vi "Traverse_Space_Server.vi"(6 "Probe Support":T1=[{"Max"=15.0, "Min"=-15.0}, {"Max"=250.0, "Min"=0.0}, {"Max"=15.0, "Min"=-15.0}] {"Min" format="%#.1f"; "Max" format="%#.1f"}, 7 "Mode":T4(ring), 8 "Entire Space":T1=[{"Max"=15001.0, "Min"=12000.0}, {"Max"=1000.0, "Min"=-1000.0}, {"Max"=700.0, "Min"=0.0}] {"Min" format="%#.1f"; "Max" format="%#.1f"}, 9 "Probe Volume":T1=[{"Max"=0.0, "Min"=0.0}, {"Max"=250.0, "Min"=0.0}, {"Max"=15.0, "Min"=-15.0}] {"Min" format="%#.1f"; "Max" format="%#.1f"}, 10 "Exclude Array":T2[](array[typedef]) {"Sizes"."Min" format="%#.1f"; "Sizes"."Max" format="%#.1f"}, 11 "Traverse Name":string) -> (0 "Entire Space Out":T1=[{"Max"=15001.0, "Min"=12000.0}, {"Max"=1000.0, "Min"=-1000.0}, {"Max"=700.0, "Min"=0.0}] {"Min" format="%#.1f"; "Max" format="%#.1f"}, 1 "Probe Volume Out":T1=[{"Max"=15.0, "Min"=-15.0}, {"Max"=250.0, "Min"=0.0}, {"Max"=15.0, "Min"=-15.0}] {"Min" format="%#.1f"; "Max" format="%#.1f"}, 2 "Exclude Array Out":T2[](array[typedef])=[{"Sizes"=[{"Max"=15000.0, "Min"=0.0}, {"Max"=1000.0, "Min"=-1000.0}, {"Max"=300.0, "Min"=0.0}], "Name"="Roughness Elements", "Exclude Type"=enum."Allow only vertical moves"}, {"Sizes"=[{"Max"=17000.0, "Min"=16000.0}, {"Max"=200.0, "Min"=-200.0}, {"Max"=-50.0, "Min"=-250.0}], "Name"="B204", "Exclude Type"=enum."Exclude completely"}] {"Sizes"."Min" format="%#.1f"; "Sizes"."Max" format="%#.1f"}, 3 "Error Comments":string, 4 "Probe Support Out":T1=[{"Max"=15.0, "Min"=-15.0}, {"Max"=250.0, "Min"=0.0}, {"Max"=15.0, "Min"=-15.0}] {"Min" format="%#.1f"; "Max" format="%#.1f"}, 5 "Space File":path)   [LabVIEW 2013]
uses:
  Gen Trav/Route mapping/Exclude_cluster.ctl
  Gen Trav/Route mapping/Box_size.ctl
  Gen Trav/Route mapping/Exclusion_type.ctl
  Globals/Constants_global.vi
panel:
  in  "Row type":string
  in  "Integer":i32
  out "Channel Values":string[][](array[string])
  # "(Relative to measurement position)"
  # "X                           Y                          Z"
  # "(Relative to measurement position)"
  # "X                           Y                          Z"
  # "X                           Y                          Z"
  # "X                           Y                          Z"
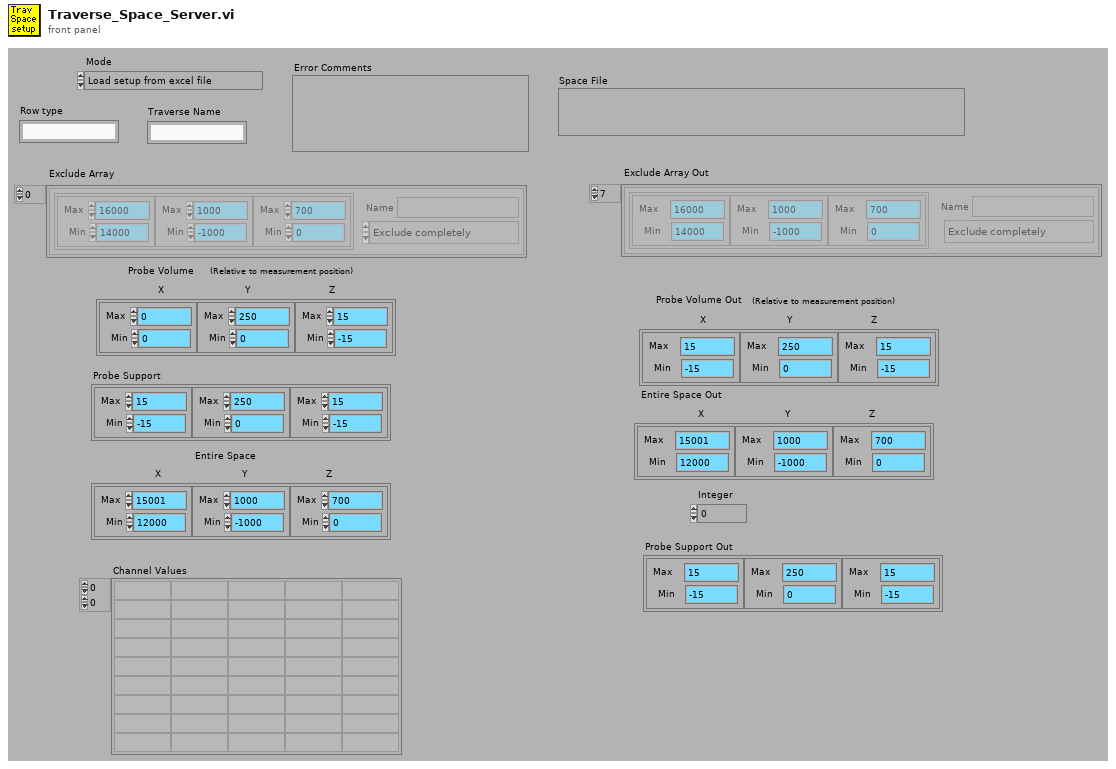
[diagram p1: front panel]
types:
  T1 = typedef "Box_size.ctl" = cluster{"Max":dbl, "Min":dbl}[]
  T2 = typedef "Exclude_cluster.ctl" = cluster{"Sizes":T1, "Name":string, "Exclude Type":T3}
  T3 = typedef "Exclusion_type.ctl" = enum16{"Exclude completely", "Allow only vertical moves"}
  T4 = enum16{"Load setup from excel file", "Save setup to excel file"}
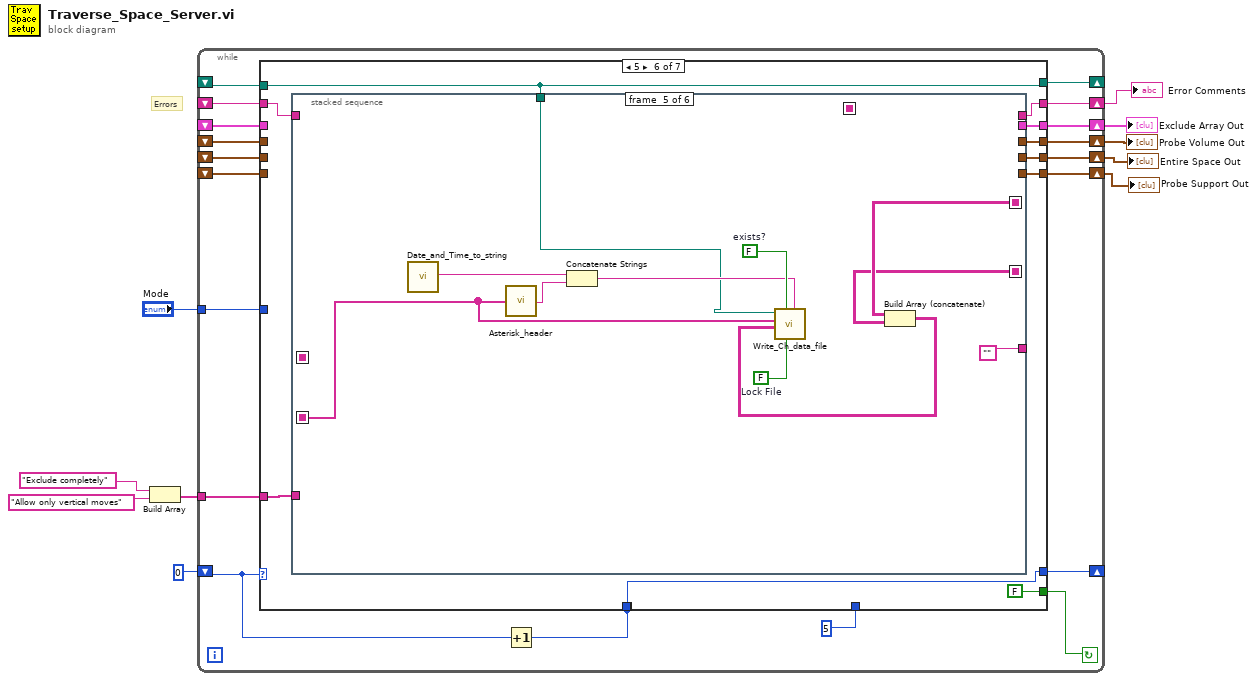
[diagram p0: block diagram]
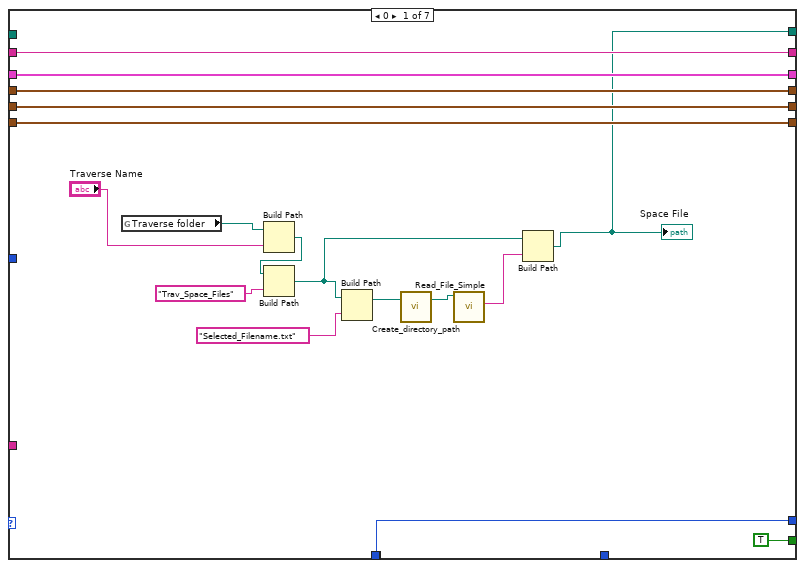
[diagram p2: hidden frame]
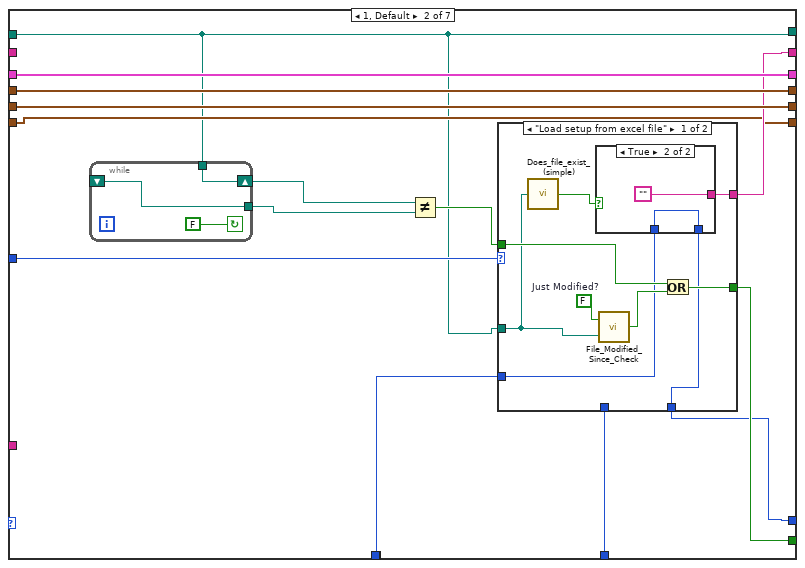
[diagram p3: hidden frame]
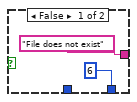
[diagram p4: hidden frame]
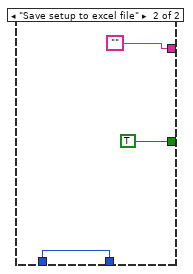
[diagram p5: hidden frame]
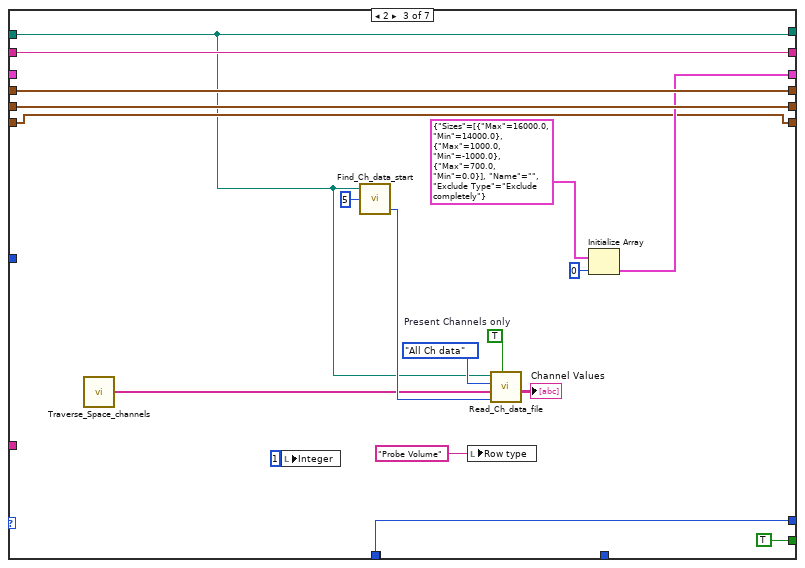
[diagram p6: hidden frame]
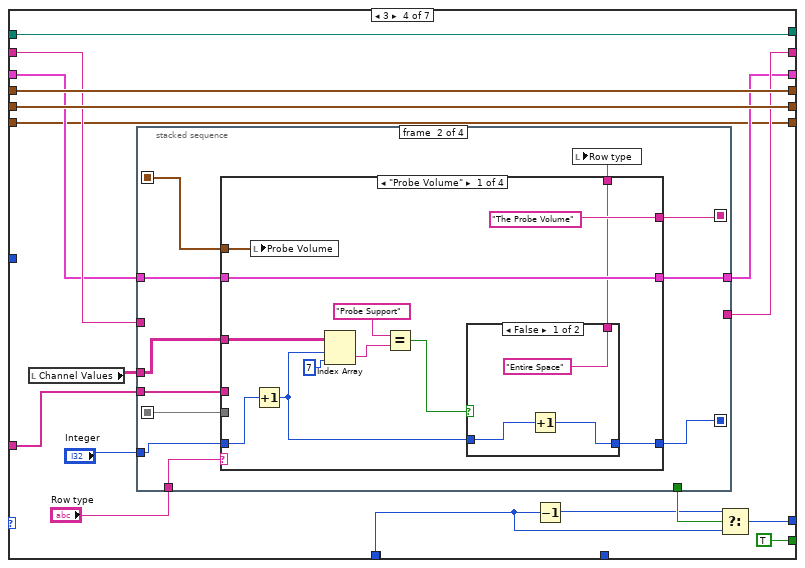
[diagram p7: hidden frame]
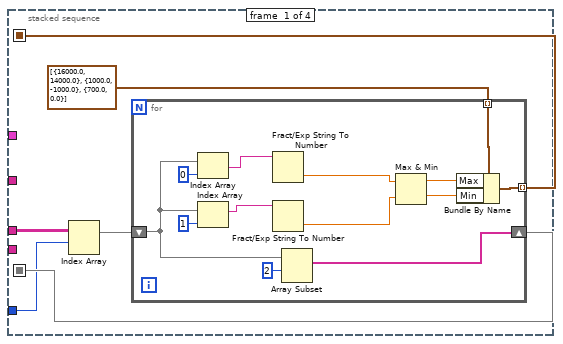
[diagram p8: hidden frame]
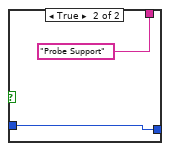
[diagram p9: hidden frame]
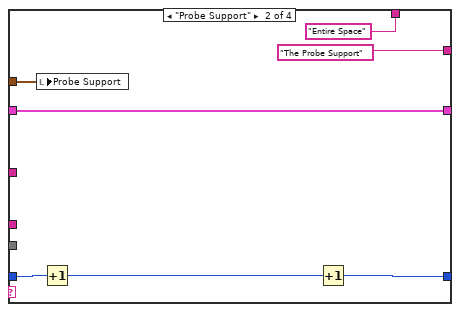
[diagram p10: hidden frame]
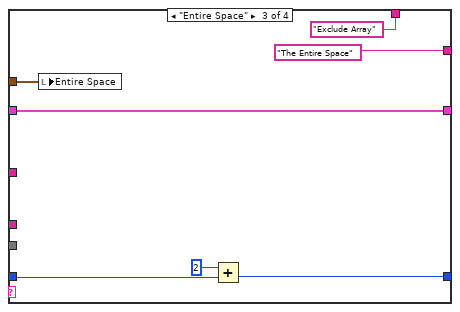
[diagram p11: hidden frame]
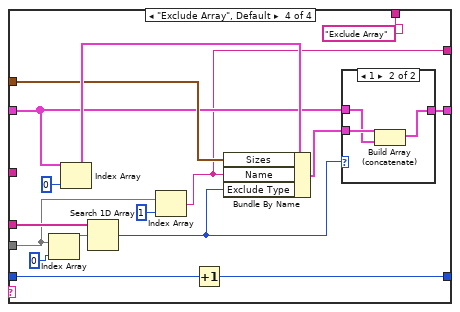
[diagram p12: hidden frame]
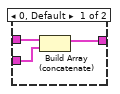
[diagram p13: hidden frame]
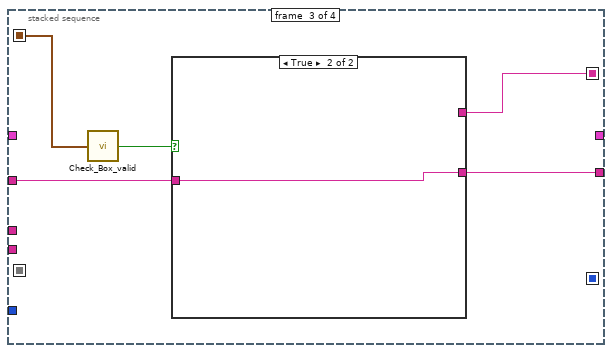
[diagram p14: hidden frame]
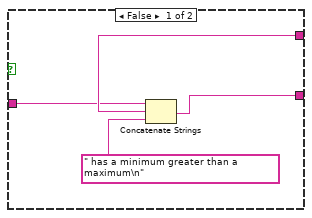
[diagram p15: hidden frame]
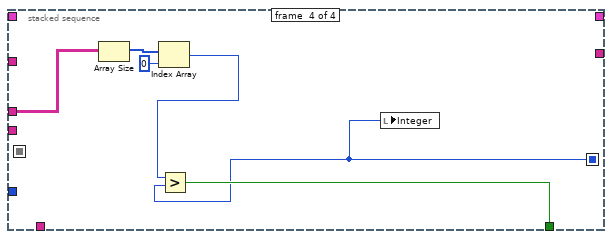
[diagram p16: hidden frame]
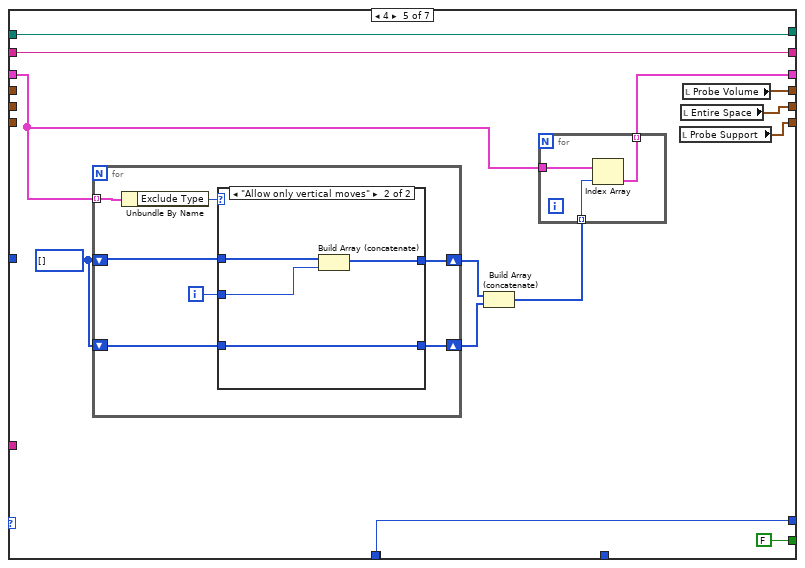
[diagram p17: hidden frame]
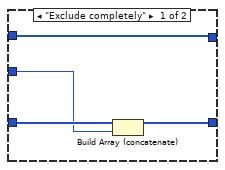
[diagram p18: hidden frame]
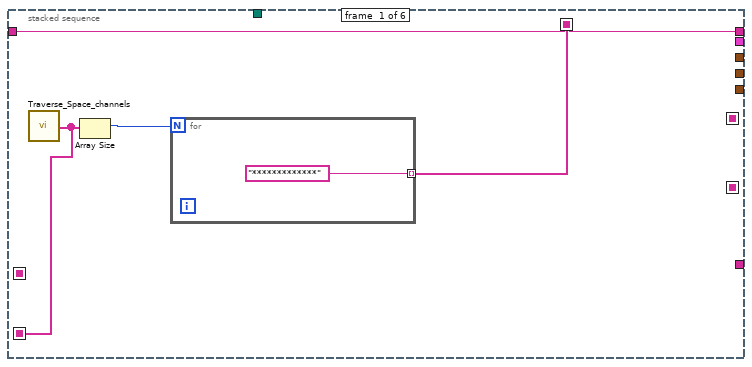
[diagram p19: hidden frame]
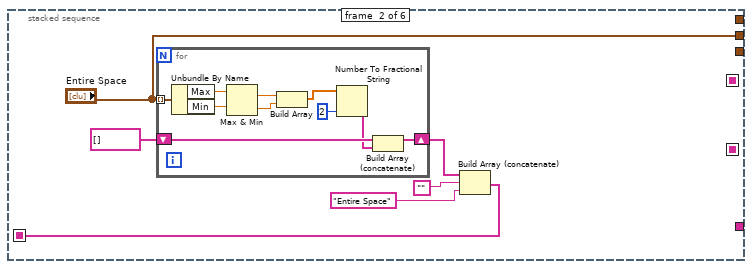
[diagram p20: hidden frame]
diagram:
  # "Errors"
  n1 = Build Array("Exclude completely", "Allow only vertical moves") -> (w4:string[])
  n2 = while {
    tunnel: w4 -> [w16]
    shift-left: _ -> [w19]
    shift-right: [w18] -> w3
    tunnel: "Mode" -> [w26]
    shift-left: _ -> [w22]
    shift-right: [w21] -> w8
    shift-left: _ -> [w24]
    shift-right: [w23] -> w2
    shift-left: _ -> [w25]
    shift-right: [w15] -> w9
    shift-left: 0 -> [w28]
    shift-right: [w27] -> _
    shift-right: [w14] -> w1
    shift-left: _ -> [w13]
    shift-right: [w12] -> _
    shift-left: _ -> [w11]
    stop <- w29 continue-if-true
    n3 = Increment(x=w28) -> (x+1=w17:i32)
    n4 = case shown="5" w28 {
      tunnel: [TRUE w52 TRUE TRUE FALSE FALSE FALSE] -> w29
      tunnel: w17 -> [w42 w56 _ _ w224 w247 w359]
      tunnel: [w42 w50 w89 w103 w224 w247 w359] -> w27
      tunnel: w26 -> [_ w60 _ _ _ _ _]
      tunnel: w25 -> [w45 w59 _ w101 w217 _ _]
      tunnel: w24 -> [w44 w58 w92 w114 _ _ _]
      tunnel: [w44 w58 w92 w114 w223 w249 w355] -> w23
      tunnel: w22 -> [w43 w57 w91 w113 _ _ _]
      tunnel: [w43 w57 w91 w113 w222 w248 w355] -> w21
      tunnel: 5 -> [_ w55 _ _ _ _ _]
      tunnel: w19 -> [w46 _ w90 w108 w225 w251 w356]
      tunnel: [w46 w51 w90 w107 w225 w252 w356] -> w18
      tunnel: w17 -> [_ _ w89 w104 _ _ _]
      tunnel: w16 -> [_ _ _ w109 _ w253 _]
      tunnel: [w45 w59 w84 w102 w216 w250 T2[] [] ("Exclude Array")] -> w15
      tunnel: [w40 w49 w82 w100 w215 w246 w355] -> w14
      tunnel: w13 -> [w40 w49 w82 w100 _ _ _]
      tunnel: [w30 w47 w80 w98 w214 w245 w354] -> w12
      tunnel: w11 -> [_ w47 w80 w98 w214 w245 w354]
      frame 0 {
        n5 = global read "Constants_global.vi" "Traverse folder"() -> (w34:path)
        n6 = Build Path(base path=w34, name or relative path="Traverse Name") -> (appended path=w36:path)
        n7 = Build Path(base path=w36, name or relative path="Trav_Space_Files" ("Substring")) -> (appended path=w32:path)
        n8 = Build Path(base path=w32, name or relative path="Selected_Filename.txt" ("Substring")) -> (appended path=w39:path)
        n9 = call "Create_directory_path.vi"("Path name"=w39) -> ("Path name Out"=w38:path)  [unwired: 1 in, 1 out]
        n10 = call "Read_File_Simple.vi"("Filename"=w38) -> ("string"=w31:string)  [unwired: 2 in, 7 out]
        n11 = Build Path(base path=w32, name or relative path=w31) -> (appended path=w30:path)
        "Space File" <- w30
      }
      frame 1, Default {
        n12 = while {
          tunnel: [w63] -> w53
          shift-left: _ -> [w63]
          shift-right: [w61] -> w54
          tunnel: w47 -> [w61]
          stop <- FALSE continue-if-true
        }
        n13 = Not Equal?(x=w54, y=w53) -> (x != y?=w48:bool)
        n14 = case shown="\"Load setup from excel file\"" w60 {
          tunnel: w47 -> [w68 _]
          tunnel: w48 -> [w71 _]
          tunnel: [w70 TRUE] -> w52
          tunnel: w56 -> [w64 _]
          tunnel: [w65 w78] -> w50
          tunnel: w55 -> [_ w78]
          tunnel: [w66 ""] -> w51
          frame "Load setup from excel file" {
            w69 = FALSE  # Just Modified?
            n15 = call "Does_file_exist_(simple).vi"("Pathname"=w68) -> ("exists?"=w67:bool)
            n16 = case shown="True" w67 {
              tunnel: ["File does not exist" ""] -> w66
              tunnel: [6 ("f") w75] -> w65
              tunnel: w64 -> [_ w75]
              frame False {
              }
              frame True {
              }
            }
            n17 = call "File_Modified_Since_Check.vi"("Pathname"=w68, "Just Modified?"=w69) -> ("Modified?"=w72:bool)
            n18 = Or(x=w71, y=w72) -> (x .or. y?=w70:bool)
          }
          frame "Save setup to excel file" {
          }
        }
      }
      frame 2 {
        w94 = TRUE  # Present Channels only
        n19 = call "Traverse_Space_channels.vi"() -> ("Channel Names"=w83:string[])
        n20 = local write "Integer"(1 ("Integer")) -> ()
        n21 = call "Find_Ch_data_start.vi"("Approx No Of Columns"=5, "Filename"=w80) -> ("Start of read offset output"=w97:i32)  [unwired: 1 in, 2 out]
        n22 = local write "Row type"("Probe Volume") -> ()
        n23 = call "Read_Ch_data_file.vi"("Present Channels only"=w94, "Start of read offset (chars.: 0)"=w97, "Present Channels"=w83, "Output"=enum16{"All Ch data", "The last few rows"}."All Ch data", "Filename"=w80) -> ("Channel Values"=→"Channel Values":string[][])  [unwired: 4 out]
        n24 = Initialize Array(T2 {"Sizes"=[{"Max"=16000.0, "Min"=14000.0}, {"Max"=1000.0, "Min"=-1000.0}, {"Max"=700.0, "Min"=0.0}], "Name"="", "Exclude Type"=enum."Exclude completely"} ("Cluster"), 0 ("Dimension Size")) -> (w84:T2[])
      }
      frame 3 {
        n25 = local read "Channel Values"() -> (w111:string[][])
        n26 = stacked-sequence {
          seq-local: [w115 _ _ _] -> [_ w144 w202 _]
          seq-local: [w117 _ _ _] -> [_ w139 _ _]
          seq-local: [_ w143 _ _] -> [_ _ w200 _]
          seq-local: [_ w137 _ _] -> [_ _ _ w208]
          tunnel: w111 -> [w120 w136 _ w210]
          tunnel: "Integer" -> [w116 w138 _ _]
          tunnel: w108 -> [_ _ w199 _]
          tunnel: [_ _ w198 _] -> w107
          tunnel: [_ w142 _ _] -> w102
          tunnel: w101 -> [_ w141 _ _]
          tunnel: w109 -> [_ w140 _ _]
          tunnel: [_ _ _ w213] -> w106
          tunnel: "Row type" -> [_ w135 _ _]
          frame #0 {
            n27 = Index Array(array=w120, index (row)=w116) -> (element=w119:string[])  [unwired: 1 in]
            n28 = for {
              shift-right: [w131] -> w117
              shift-left: w119 -> [w130]
              tunnel: T1 [{"Max"=16000.0, "Min"=14000.0}, {"Max"=1000.0, "Min"=-1000.0}, {"Max"=700.0, "Min"=0.0}] ("Entire Space") -> [w126] mode=indexing
              tunnel: [w125] -> w115 mode=indexing
              n29 = Index Array(array=w130, index=0 ("Index")) -> (element=w128:string)
              n30 = Index Array(array=w130, index=1 ("Index")) -> (element=w127:string)
              n31 = Fract/Exp String To Number(string=w128) -> (number=w124:dbl)  [unwired: 4 out]
              n32 = Fract/Exp String To Number(string=w127) -> (number=w123:dbl)  [unwired: 4 out]
              n33 = Array Subset(array=w130, index=2 ("Array Index")) -> (w131:string[])  [unwired: 1 in]
              n34 = Max & Min(x=w124, y=w123) -> (max(x,y)=w122:dbl, min(x,y)=w121:dbl)
              n35 = Bundle By Name(cluster=w126, "Max"=w122, "Min"=w121) -> (w125:cluster{"Max":dbl, "Min":dbl})
            }
          }
          frame #1 {
            n36 = case shown="\"Probe Volume\"" w135 {
              tunnel: w144 -> [w153 w165 w170 w189]
              tunnel: ["The Probe Volume" "The Probe Support" "The Entire Space" w180] -> w143
              tunnel: [w155 w167 w174 w188] -> w142
              tunnel: w141 -> [w155 w167 w174 w186]
              tunnel: w140 -> [_ _ _ w185]
              tunnel: w139 -> [_ _ _ w181]
              tunnel: w138 -> [w152 w164 w172 w179]
              tunnel: [w154 w166 w171 w178] -> w137
              tunnel: w136 -> [w151 _ _ _]
              tunnel: [w145 "Entire Space" "Exclude Array" "Exclude Array"] -> w134
              frame "Probe Volume" {
                n37 = local write "Probe Volume"(w153) -> ()
                n38 = Increment(x=w152) -> (x+1=w146:i32)
                n39 = Index Array(array=w151, index (row)=w146, index (col)=7 ("disabled index (col)")) -> (element=w149:string)
                n40 = Equal?(x="Probe Support", y=w149) -> (x = y?=w147:bool)
                n41 = case shown="False" w147 {
                  tunnel: [w158 w161] -> w154
                  tunnel: w146 -> [w159 w161]
                  tunnel: ["Entire Space" "Probe Support"] -> w145
                  frame False {
                    n42 = Increment(x=w159) -> (x+1=w158:i32)
                  }
                  frame True {
                  }
                }
              }
              frame "Probe Support" {
                n43 = local write "Probe Support"(w165) -> ()
                n44 = Increment(x=w164) -> (x+1=w163:i32)
                n45 = Increment(x=w163) -> (x+1=w166:i32)
              }
              frame "Entire Space" {
                n46 = local write "Entire Space"(w170) -> ()
                n47 = Add(x=2, y=w172) -> (x+y=w171:i32)
              }
              frame "Exclude Array", Default {
                n48 = Index Array(array=w181, index=0 ("Index")) -> (element=w183:string)
                n49 = Index Array(array=w186, index=0 ("Index")) -> (element=w190:T2)
                n50 = Search 1D Array(1D array=w185, element=w183) -> (index of element=w177:i32)  [unwired: 1 out]
                n51 = Index Array(array=w181, index=1 ("Index")) -> (element=w180:string)
                n52 = Increment(x=w179) -> (x+1=w178:i32)
                n53 = Bundle By Name(cluster=w190, "Sizes"=w189, "Name"=w180, "Exclude Type"=w177) -> (w187:T2)
                n54 = case shown="1" w177 {
                  tunnel: [w194 w195] -> w188
                  tunnel: w187 -> [w193 w197]
                  tunnel: w186 -> [w192 w196]
                  frame 0, Default {
                    n55 = Build Array (concatenate)(w192, w193) -> (w194:T2[])
                  }
                  frame 1 {
                    n56 = Build Array (concatenate)(w197, w196) -> (w195:T2[])
                  }
                }
              }
            }
            n57 = local write "Row type"(w134) -> ()
          }
          frame #2 {
            n58 = call "Check_Box_valid.vi"("Box to check"=w202) -> ("Valid Box"=w201:bool)
            n59 = case shown="True" w201 {
              tunnel: w200 -> [w205 _]
              tunnel: w199 -> [w204 w207]
              tunnel: [w203 w207] -> w198
              frame False {
                n60 = Concatenate Strings(w204, w205, " has a minimum greater than a maximum\n") -> (w203:string)
              }
              frame True {
              }
            }
          }
          frame #3 {
            n61 = Array Size(array=w210) -> (size(s)=w211:i32[])
            n62 = Index Array(array=w211, index=0 ("Index")) -> (element=w209:i32)
            n63 = Greater?(x=w209, y=w208) -> (0:w213:bool)
            n64 = local write "Integer"(w208) -> ()
          }
        }
        n65 = Decrement(x=w104) -> (x-1=w105:i32)
        n66 = Select(t=w105, s=w106, f=w104) -> (s? t:f=w103:i32)
      }
      frame 4 {
        w221 = i32[] []
        n67 = for {
          tunnel: w217 -> [w230] mode=indexing
          shift-right: [w234] -> w219
          shift-left: w221 -> [w235]
          shift-right: [w233] -> w220
          shift-left: w221 -> [w232]
          i -> [w231]
          n68 = Unbundle By Name(w230) -> ("Exclude Type"=w236:T3)
          n69 = case shown="\"Allow only vertical moves\"" w236 {
            tunnel: w235 -> [w238 w244]
            tunnel: [w238 w243] -> w234
            tunnel: [w239 w242] -> w233
            tunnel: w232 -> [w240 w242]
            tunnel: w231 -> [w237 w241]
            frame "Exclude completely" {
              n70 = Build Array (concatenate)(w240, w237) -> (w239:i32[])
            }
            frame "Allow only vertical moves" {
              n71 = Build Array (concatenate)(w244, w241) -> (w243:i32[])
            }
          }
        }
        n72 = Build Array (concatenate)(w219, w220) -> (w218:i32[])
        n73 = for {
          tunnel: w218 -> [w229] mode=indexing
          tunnel: w217 -> [w228]
          tunnel: [w227] -> w216 mode=indexing
          n74 = Index Array(array=w228, index=w229) -> (element=w227:T2)
        }
        n75 = local read "Probe Support"() -> (w215:T1)
        n76 = local read "Entire Space"() -> (w222:T1)
        n77 = local read "Probe Volume"() -> (w223:T1)
      }
      frame 5 {
        n78 = stacked-sequence {
          seq-local: [_ _ _ w312 _ _] -> [_ _ _ _ w337 _]
          seq-local: [_ _ w288 _ _ _] -> [_ _ _ _ w338 _]
          seq-local: [w257 _ _ _ _ _] -> [_ _ w277 _ _ _]
          seq-local: [w255 _ _ _ _ _] -> [_ _ _ _ w333 _]
          seq-local: [_ w261 _ _ _ _] -> [_ _ w278 _ _ _]
          tunnel: [_ _ _ _ "" _] -> _
          tunnel: w253 -> [_ _ _ w311 _ _]
          tunnel: [w256 _ _ _ _ _] -> w252
          tunnel: w251 -> [w256 _ _ _ _ _]
          tunnel: [_ _ _ "Exclude Array" _ _] -> w250
          tunnel: [_ _ "Probe Volume" _ _ _] -> w249
          tunnel: [_ "Entire Space" _ _ _ _] -> w248
          tunnel: w245 -> [_ _ _ _ w332 w347]
          tunnel: [_ _ "Probe Support" _ _ _] -> w246
          frame #0 {
            n79 = call "Traverse_Space_channels.vi"() -> ("Channel Names"=w255:string[])
            n80 = Array Size(array=w255) -> (size(s)=w258:i32)
            n81 = for {
              N: w258 -> [_]
              tunnel: ["*************"] -> w257 mode=indexing
            }
          }
          frame #1 {
            n82 = for {
              shift-right: [w271] -> w264
              shift-left: string[] [] -> [w273]
              tunnel: "Entire Space" -> [w268] mode=indexing
              n83 = Unbundle By Name(w268) -> ("Max"=w267:dbl, "Min"=w266:dbl)
              n84 = Max & Min(x=w267, y=w266) -> (max(x,y)=w270:dbl, min(x,y)=w269:dbl)
              n85 = Build Array(w270, w269) -> (w275:dbl[])
              n86 = Number To Fractional String(number=w275, precision (6)=i16 2) -> (F-format string=w272:string[])  [unwired: 2 out]
              n87 = Build Array (concatenate)(w273, w272) -> (w271:string[])
            }
            n88 = Build Array (concatenate)(w264, "", "Entire Space" ("Input Element")) -> (w261:string[])
          }
          frame #2 {
            w289 = string[] []
            n89 = for {
              tunnel: "Probe Volume" -> [w309] mode=indexing
              shift-right: [w304] -> w287
              shift-left: w289 -> [w306]
              n90 = Unbundle By Name(w309) -> ("Max"=w303:dbl, "Min"=w302:dbl)
              n91 = Max & Min(x=w303, y=w302) -> (max(x,y)=w301:dbl, min(x,y)=w300:dbl)
              n92 = Build Array(w301, w300) -> (w308:dbl[])
              n93 = Number To Fractional String(number=w308, precision (6)=i16 2) -> (F-format string=w305:string[])  [unwired: 2 out]
              n94 = Build Array (concatenate)(w306, w305) -> (w304:string[])
            }
            n95 = for {
              tunnel: "Probe Support" -> [w299] mode=indexing
              shift-right: [w294] -> w282
              shift-left: w289 -> [w296]
              n96 = Unbundle By Name(w299) -> ("Max"=w293:dbl, "Min"=w292:dbl)
              n97 = Max & Min(x=w293, y=w292) -> (max(x,y)=w291:dbl, min(x,y)=w290:dbl)
              n98 = Build Array(w291, w290) -> (w298:dbl[])
              n99 = Number To Fractional String(number=w298, precision (6)=i16 2) -> (F-format string=w295:string[])  [unwired: 2 out]
              n100 = Build Array (concatenate)(w296, w295) -> (w294:string[])
            }
            n101 = Build Array (concatenate)(w287, "", "Probe Volume" ("Input Element")) -> (w281:string[])
            n102 = Build Array (concatenate)(w282, "", "Probe Support" ("Input Element")) -> (w279:string[])
            n103 = Build Array(w277, w281, w279, w277, w278, w277) -> (w288:string[][])
          }
          frame #3 {
            n104 = for {
              tunnel: "Exclude Array" -> [w319] mode=indexing
              tunnel: w311 -> [w317]
              tunnel: [w313] -> w312 mode=indexing
              n105 = Unbundle By Name(w319) -> ("Sizes"=w321:T1)
              n106 = Unbundle By Name(w319) -> ("Exclude Type"=w318:T3, "Name"=w314:string)
              n107 = for {
                tunnel: w321 -> [w331] mode=indexing
                shift-right: [w326] -> w316
                shift-left: string[] [] -> [w328]
                n108 = Unbundle By Name(w331) -> ("Max"=w325:dbl, "Min"=w324:dbl)
                n109 = Max & Min(x=w325, y=w324) -> (max(x,y)=w323:dbl, min(x,y)=w322:dbl)
                n110 = Build Array(w323, w322) -> (w330:dbl[])
                n111 = Number To Fractional String(number=w330, precision (6)=i16 2) -> (F-format string=w327:string[])  [unwired: 2 out]
                n112 = Build Array (concatenate)(w328, w327) -> (w326:string[])
              }
              n113 = Index Array(array=w317, index=w318) -> (element=w315:string)
              n114 = Build Array (concatenate)(w316, w315, w314) -> (w313:string[])
            }
          }
          frame #4 {
            w334 = FALSE  # Lock File
            w342 = FALSE  # exists?
            n115 = call "Date_and_Time_to_string.vi"() -> ("Date and time (spreadsheet)"=w339:string)
            n116 = call "Asterisk_header.vi"("Channel names"=w333) -> ("Header string"=w341:string)
            n117 = Concatenate Strings(w339, w341) -> (w340:string)
            n118 = Build Array (concatenate)(w338, w337) -> (w336:string[][])
            n119 = call "Write_Ch_data_file.vi"("Header string"=w340, "Lock File"=w334, "exists?"=w342, "Channel Values"=w336, "Channel names"=w333, "Filename"=w332) -> ()  [unwired: 2 in, 4 out]
          }
          frame #5 {
            n120 = Strip Path(path=w347) -> (name=w346:string)  [unwired: 1 out]
            n121 = call "Create_Error_log_folders.vi"("Log Folder"="Traverse_Space_files", "Log Filename"=w346) -> ("exists?"=w349:bool, "Local Log File"=w348:path)  [unwired: 1 in, 1 out]
            n122 = case shown="True" w349 {
              tunnel: [w351 w353] -> w345
              tunnel: w348 -> [w351 w352]
              frame False {
              }
              frame True {
                n123 = call "Find_Unique_Filename.vi"("Path In"=w352) -> ("Unique Path Out"=w353:path)  [unwired: 1 in, 1 out]
              }
            }
            n124 = call "Create_directory_path.vi"("Path name"=w345) -> ("error out"=w343:errorcluster, "Path name Out"=w344:path)  [unwired: 1 in]
            n125 = Copy(8:w343, 10:w344, 11:w347) -> ()  [unwired: 5 out]
          }
        }
      }
      frame 6 {
        w355 = T1 [] ("Probe Volume")
      }
    }
  }
  "Error Comments" <- w3
  "Probe Volume Out" <- w2
  "Entire Space Out" <- w8
  "Exclude Array Out" <- w9
  "Probe Support Out" <- w1
